vi "PositionPID.vi"() -> ()   [LabVIEW 2016]
uses:
  <vilib>/MakerHub/LINX/Public/Utilities/Open Serial.vi
  <vilib>/addons/control/pid/pid.llb/PID (DBL).vi
  <vilib>/MakerHub/LINX/LMH-LINX.lvlib
  <vilib>/addons/control/pid/NI_PID_pid.lvlib
panel:
  in  "T":u32
  in  "PID gains":T1={"proportional gain (Kc)"=1.0, "integral time (Ti, min)"=0.01, "derivative time (Td, min)"=0.0} {"derivative time (Td, min)" format="%.3f"; "integral time (Ti, min)" format="%.3f"; "proportional gain (Kc)" format="%.3f"}
  in  "output range":cluster{"output high":dbl, "output low":dbl}={"output high"=100.0, "output low"=-100.0} {"output low" format="%.2f"; "output high" format="%.2f"}
  out "Set-Point - Position":dynamicdata(graph)
  out "Voltage":dbl(graph)
  out "Loop Rate (Hz)":u32
  in  "IN 4":u8
  in  "IN3":u8
  in  "PWM Channel":u8
  in  "stop":bool
  in  "Source Voltage":dbl
  in  "setpoint":dbl format="%.2f"
  in  "Number Of Pulses":i32
  in  "Serial Port":refnum<visa-resource-name>="N/A"
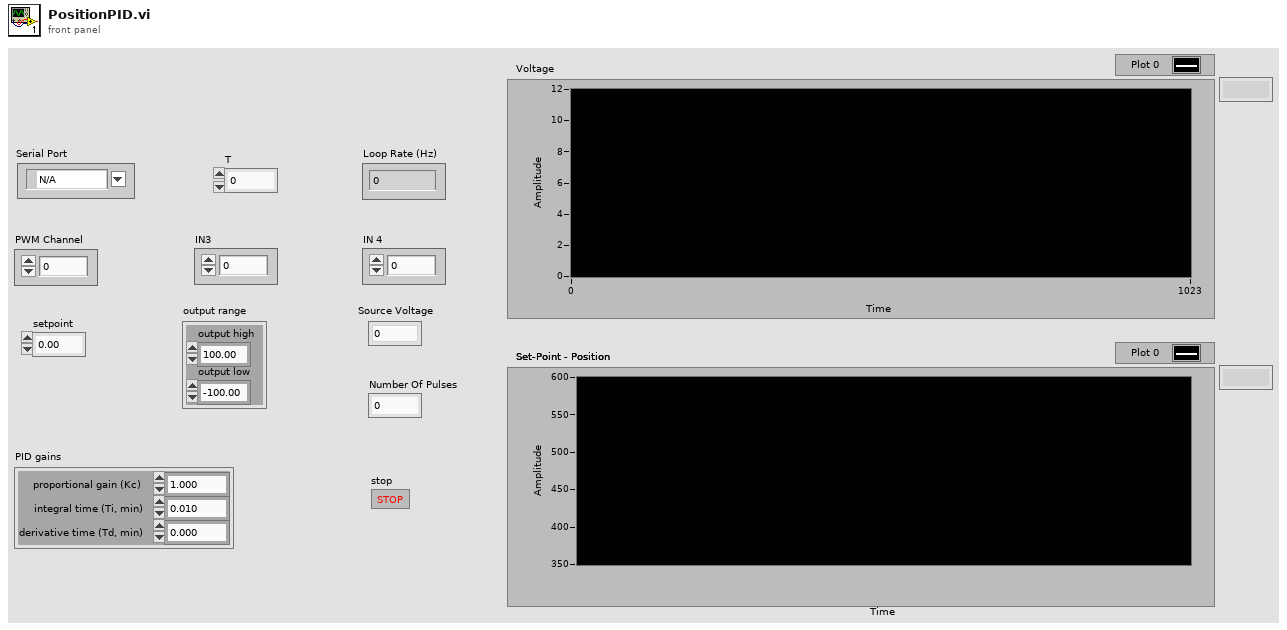
[diagram p1: front panel]
types:
  T1 = cluster{"proportional gain (Kc)":dbl, "integral time (Ti, min)":dbl, "derivative time (Td, min)":dbl}
  T2 = typedef "LMH-LINX.lvlib/LINX Ref.ctl" = cluster{"IO":T3, "Interface":T4, "LINX Device Config":T5}
  T3 = typedef "LMH-LINX.lvlib/Platform.ctl" = enum16{"Remote", "Local"}
  T4 = typedef "LMH-LINX.lvlib/Interface.ctl" = enum16{"Serial", "TCP"}
  T5 = typedef "LMH-LINX.lvlib/Device.lvlib/LINX Device Config.ctl" = cluster{"Interface":T4, "COM Port":refnum<visa-resource-name>, "TCP Configuration":T6, "Device Family":u8, "Device ID":u8, "Device Name":string, "TCP Ref":refnum<k5>, "Channels":T7}
  T6 = typedef "LMH-LINX.lvlib/Device.lvlib/TCP Config.ctl" = cluster{"IP Address":string, "Port":u16}
  T7 = typedef "LMH-LINX.lvlib/Channels.ctl" = cluster{"DI":u8[], "DO":u8[], "AI":u8[], "AO":u8[], "PWM":u8[], "QE":u8[], "UART":u8[], "I2C 2":u8[], "SPI":u8[], "CAN":u8[], "Servo":u8[], "AI Ref (V)":dbl, "AI Resolution (Bits)":u8, "AO Ref (V)":dbl, "AO Resolution (Bits)":u8}
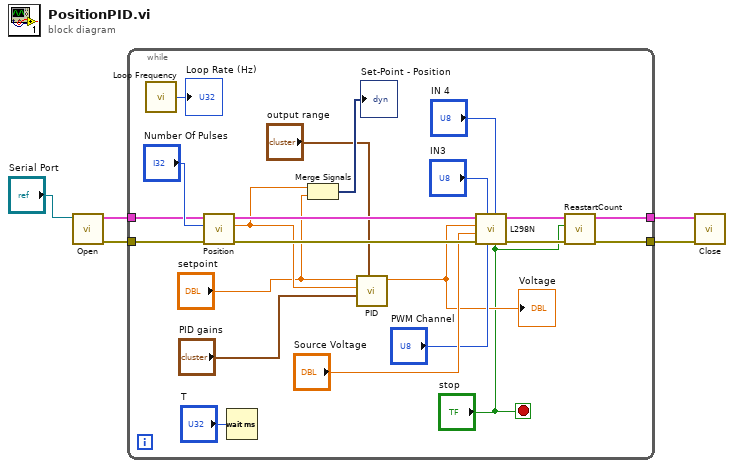
[diagram p0: block diagram]
diagram:
  n1 = call-poly <vilib>:"Open.vi"("Serial Port"="Serial Port") -> ("Error Out"=w4:errorcluster, "LINX Resource"=w5:T2)  [unwired: 8 in, 1 out]
  n2 = while {
    tunnel: w5 -> [w26]
    tunnel: w4 -> [w25]
    tunnel: [w9] -> w3
    tunnel: [w10] -> w2
    stop <- "stop" stop-if-true
    n3 = call <vilib>:"Loop Frequency.vi"() -> ("Loop Rate (Hz)"=→"Loop Rate (Hz)":u32)
    n4 = call "Position.vi"("Error In"=w25, "Number of pulses"="Number Of Pulses", "LINX Resource IN"=w26) -> ("Error Out"=w23:errorcluster, "Position (Degrees)"=w16:dbl, "LINX Resource OUT"=w24:T2)  [unwired: 6 in]
    n5 = Wait (ms)(milliseconds to wait="T") -> ()  [unwired: 1 out]
    n6 = Merge Signals(w16, "setpoint") -> (→"Set-Point - Position":dynamicdata)
    n7 = call-poly <vilib>:"PID.vi"("output range"="output range", "PID gains"="PID gains", "process variable"=w16, "setpoint"="setpoint") -> ("output"=w17:dbl)  [unwired: 6 in, 1 out]
    "Voltage" <- w17
    n8 = call "L298N.vi"("Turn Off"="stop", "IN 4"="IN 4", "PWM Channel"="PWM Channel", "IN3"="IN3", "Error In"=w23, "Source Voltage"="Source Voltage", "Voltage"=w17, "LINX Resource IN"=w24) -> ("Error Out"=w7:errorcluster, "LINX Resource OUT"=w8:T2)  [unwired: 2 in]
    n9 = call "ReastartCount.vi"("Error In"=w7, "Activate"="stop", "LINX Resource IN"=w8) -> ("Error Out"=w10:errorcluster, "LINX Resource OUT"=w9:T2)  [unwired: 7 in]
  }
  n10 = call <vilib>:"Close.vi"("Error In"=w2, "LINX Resource"=w3) -> ()  [unwired: 9 in, 1 out]
